vi "Set_file_name.vi"() -> (2 "appended path":path)   [LabVIEW 2017]
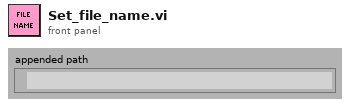
[diagram p1: front panel]
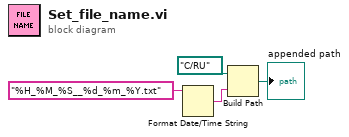
[diagram p0: block diagram]
diagram:
  n1 = Format Date/Time String(time format string (%c)="%H_%M_%S__%d_%m_%Y.txt") -> (date/time string=w2:string)  [unwired: 2 in]
  n2 = Build Path(base path=path "C:/RU" ("file"), name or relative path=w2) -> (appended path=→"appended path":path)
